vi "EF_CommonAverageRef.vi"(1 "Array Of Waveforms in":waveform(dbl)[](array[waveform])) -> (0 "Array Waveforms out":waveform(dbl)[](array[waveform]))   [LabVIEW 2016, in "Feature Extraction.lvlib"]
uses:
  Feature Extraction.lvlib
panel:
  # "This VI is a part of BCI Design library, http://www.ru-bci.org \nCopyright © 2020, Sotnikov Peter, All rights reserved. License: GNU GPLv3"
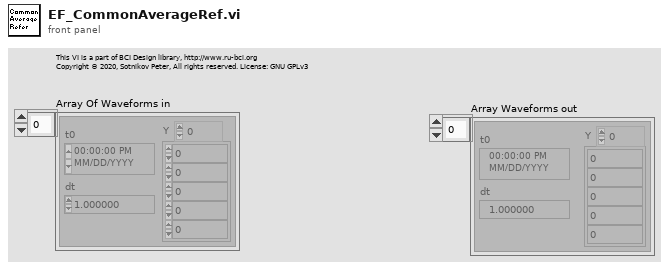
[diagram p1: front panel]
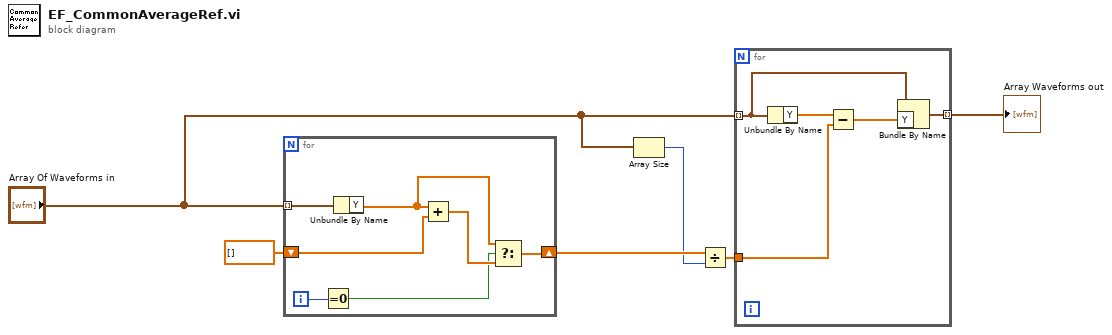
[diagram p0: block diagram]
diagram:
  n1 = for {
    tunnel: "Array Of Waveforms in" -> [w13] mode=indexing
    shift-right: [w10] -> w5
    shift-left: dbl[] [] ("Y") -> [w12]
    i -> [w9]
    n2 = Equal To 0?(x=w9) -> (x = 0?=w8:bool)
    n3 = Unbundle By Name(w13) -> ("Y"=w7:dbl[])
    n4 = Add(x=w7, y=w12) -> (x+y=w11:dbl[])
    n5 = Select(t=w7, s=w8, f=w11) -> (s? t:f=w10:dbl[])
  }
  n6 = Array Size(array="Array Of Waveforms in") -> (size(s)=w1:i32)
  n7 = Divide(x=w5, y=w1) -> (x/y=w4:dbl[])
  n8 = for {
    tunnel: "Array Of Waveforms in" -> [w16] mode=indexing
    tunnel: w4 -> [w17]
    tunnel: [w14] -> w3 mode=indexing
    n9 = Unbundle By Name(w16) -> ("Y"=w18:dbl[])
    n10 = Subtract(x=w18, y=w17) -> (x-y=w15:dbl[])
    n11 = Bundle By Name(cluster=w16, "Y"=w15) -> (w14:waveform(dbl))
  }
  "Array Waveforms out" <- w3
